vi "SectionMap_FGV.vi"(6 "Sections":string[](array[string]), 8 "error in":errorcluster, 9 "Action":T1=enum."Filter Valid Nodes", 10 "Child Section Name":string, 11 "Parent Section Name":string) -> (0 "error out":errorcluster, 3 "Invalid Child Sections":string[](array[string]))   [LabVIEW 2025]
uses:
  Types/Section Map Action.ctl
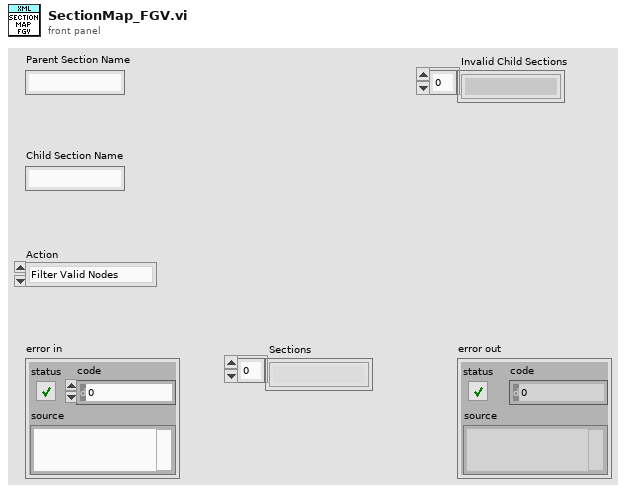
[diagram p1: front panel]
types:
  T1 = typedef "Section Map Action.ctl" = enum16{"Delete Child Node", "Filter Valid Nodes", "Add Child Section", "Initialize"}
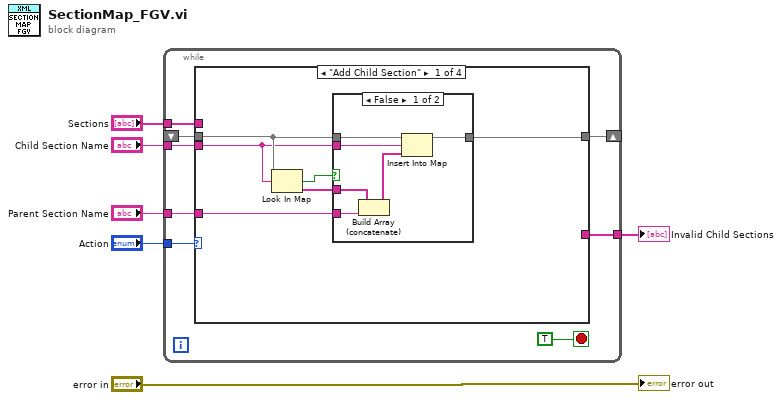
[diagram p0: block diagram]
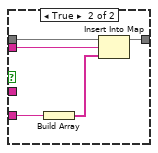
[diagram p2: hidden frame]
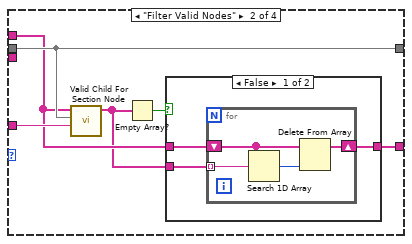
[diagram p3: hidden frame]
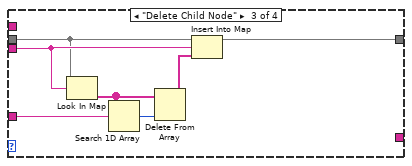
[diagram p5: hidden frame]
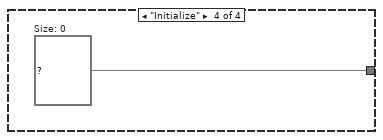
[diagram p6: hidden frame]
diagram:
  n1 = while {
    shift-right: [w14] -> _
    shift-left: _ -> [w11]
    tunnel: "Action" -> [w12]
    tunnel: "Child Section Name" -> [w10]
    tunnel: "Parent Section Name" -> [w9]
    tunnel: "Sections" -> [w8]
    tunnel: [w7] -> w2
    stop <- TRUE stop-if-true
    n2 = case shown="\"Add Child Section\"" w12 {
      tunnel: [w16 w37 w46 w53] -> w14
      tunnel: w11 -> [w19 w37 w48 _]
      tunnel: w10 -> [w18 _ w49 _]
      tunnel: w9 -> [w17 w36 w52 _]
      tunnel: w8 -> [_ w35 _ _]
      tunnel: [_ w34 _ _] -> w7
      frame "Add Child Section" {
        n3 = Look In Map(map=w19, key=w18) -> (key not found?=w20:bool, value=w15:string[])  [unwired: 1 in]
        n4 = case shown="False" w20 {
          tunnel: w19 -> [w26 w31]
          tunnel: w18 -> [w21 w30]
          tunnel: w17 -> [w23 w29]
          tunnel: [w22 w27] -> w16
          tunnel: w15 -> [w24 _]
          frame False {
            n5 = Build Array (concatenate)(w24, w23) -> (w25:string[])
            n6 = Insert Into Map(map in=w26, key=w21, value=w25) -> (map out=w22:map{string, string[]})  [unwired: 2 out]
          }
          frame True {
            n7 = Build Array(w29) -> (w28:string[])
            n8 = Insert Into Map(map in=w31, key=w30, value=w28) -> (map out=w27:map{string, string[]})  [unwired: 2 out]
          }
        }
      }
      frame "Filter Valid Nodes" {
        n9 = call "Valid Child For Section Node.vi"("Section Name"=w36, "Map"=w37, "Sections"=w35) -> ("Invalid Child Sections"=w32:string[])  [unwired: 8 in]
        n10 = Empty Array?(array=w32) -> (empty?=w33:bool)
        n11 = case shown="False" w33 {
          tunnel: w32 -> [w40 _]
          tunnel: w35 -> [w38 w45]
          tunnel: [w39 w45] -> w34
          frame False {
            n12 = for {
              tunnel: w40 -> [w44] mode=indexing
              shift-right: [w41] -> w39
              shift-left: w38 -> [w42]
              n13 = Search 1D Array(1D array=w42, element=w44) -> (index of element=w43:i32)  [unwired: 1 in]
              n14 = Delete From Array(array=w42, index=w43) -> (array with subset deleted=w41:string[])  [unwired: 1 in, 1 out]
            }
          }
          frame True {
          }
        }
      }
      frame "Delete Child Node" {
        n15 = Look In Map(map=w48, key=w49) -> (value=w51:string[])  [unwired: 1 in, 1 out]
        n16 = Search 1D Array(1D array=w51, element=w52) -> (index of element=w50:i32)  [unwired: 1 in]
        n17 = Delete From Array(array=w51, index=w50) -> (array with subset deleted=w47:string[])  [unwired: 1 in, 1 out]
        n18 = Insert Into Map(map in=w48, key=w49, value=w47) -> (map out=w46:map{string, string[]})  [unwired: 2 out]
      }
      frame "Initialize" {
        w53 = map{string, string[]} {}  # Size: 0
      }
    }
  }
  "Invalid Child Sections" <- w2
  "error out" <- "error in"
